vi "MQTT_Simple_Connect_and_Publish.vi"() -> ()   [LabVIEW 2018, in "MQTT_Functions.lvlib"]
uses:
  MQTT_Functions.lvlib
  Controls/QoS.ctl
  Controls/Retain_Flag.ctl
  Controls/DUP_Flag.ctl
  Controls/Connection_Return_Codes.ctl
  Controls/User_Info.ctl
  Controls/Connect_Flags.ctl
panel:
  in  "User Info":T1
  out "Message published":string
  in  "Stop Publishing":bool
  out "Message ID (acknowledged)":u16=10
  out "Acknowledged":bool
  in  "Message ID":u16=20
  in  "MQTT Broker":cluster{"address (IP)":string, "port":u16}={"address (IP)"="127.0.0.1", "port"=1883}
  in  "Message to be published":string="Quaxo says it's "
  out "Connection Status":T2=enum."Connection refused: not authorized"
  out "error out":errorcluster
  in  "Client ID":string="NodeE-12345"
  in  "error in (no error)":errorcluster
  in  "Topic":string[](array[string])
  in  "Publish Meta":cluster{"QoS":T3, "Retain":T4, "DUP":T5}
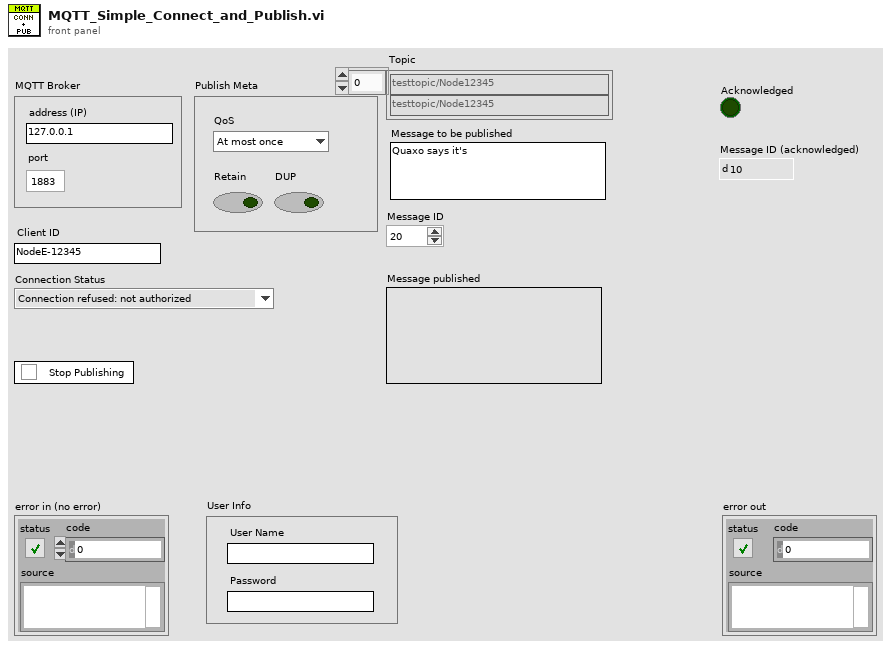
[diagram p1: front panel]
types:
  T1 = typedef "MQTT_Functions.lvlib/User_Info.ctl" = cluster{"User Name":string, "Password":string}
  T2 = typedef "MQTT_Functions.lvlib/Connection_Return_Codes.ctl" = enum16{"Connection accepted", "Connection refused: unacceptable protocol version", "Connection refused: identifier rejected", "Connection refused: Server unavailable", "Connection refused: bad user name or password", "Connection refused: not authorized"}
  T3 = typedef "MQTT_Functions.lvlib/QoS.ctl" = enum8{"At most once", "At least once", "Exactly once", "Reserved"}
  T4 = typedef "MQTT_Functions.lvlib/Retain_Flag.ctl" = bool
  T5 = typedef "MQTT_Functions.lvlib/DUP_Flag.ctl" = bool
  T6 = typedef "MQTT_Functions.lvlib/Connect_Flags.ctl" = cluster{"user name":bool, "password":bool, "will retain":bool, "will flag":bool, "clean session":bool, "reserved":bool, "will QoS":T3}
  T7 = cluster{"QoS":T3, "DUP":T5, "Retain":T4, "Keep Alive (sec)":u16}
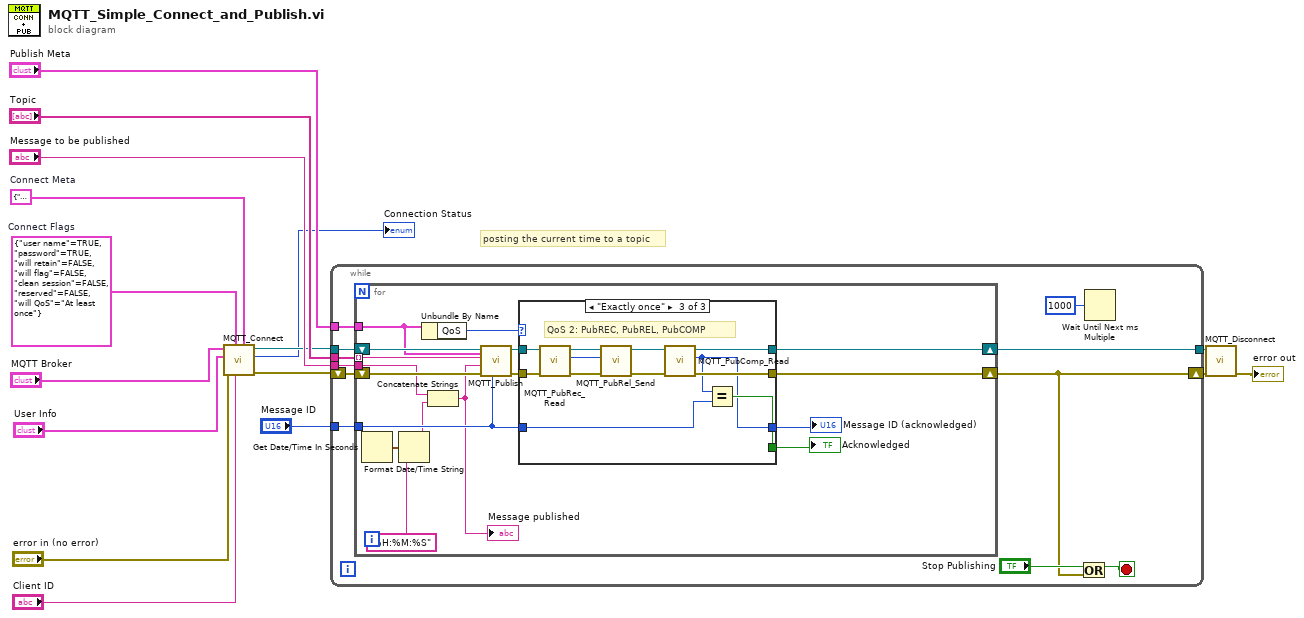
[diagram p0: block diagram]
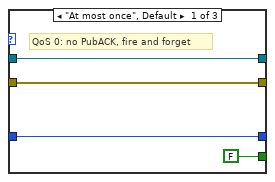
[diagram p2: hidden frame]
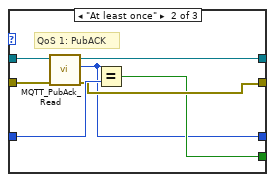
[diagram p3: hidden frame]
diagram:
  w14 = T6 {"user name"=TRUE, "password"=TRUE, "will retain"=FALSE, "will flag"=FALSE, "clean session"=FALSE, "reserved"=FALSE, "will QoS"=enum."At least once"}  # Connect Flags
  w11 = T7 {"QoS"=enum."At most once", "DUP"=FALSE, "Retain"=FALSE, "Keep Alive (sec)"=60}  # Connect Meta
  # "posting the current time to a topic"
  n1 = call "MQTT_Connect.vi"("Connect Meta"=w11, "Client ID"="Client ID", "Connect Flags"=w14, "error in (no error)"="error in (no error)", "User Info"="User Info", "MQTT Broker"="MQTT Broker") -> ("error out"=w2:errorcluster, "Connection Status"=→"Connection Status":T2, "connection ID out"=w4:refnum<k5>)  [unwired: 3 in]
  n2 = while {
    tunnel: "Topic" -> [w27]
    tunnel: "Message to be published" -> [w20]
    tunnel: w4 -> [w26]
    tunnel: "Publish Meta" -> [w24]
    tunnel: [w23] -> w7
    tunnel: "Message ID" -> [w22]
    shift-right: [w18] -> w8
    shift-left: w2 -> [w25]
    stop <- w19 stop-if-true
    n3 = for {
      tunnel: w27 -> [w44] mode=indexing
      tunnel: w24 -> [w41]
      tunnel: w22 -> [w36]
      tunnel: w20 -> [w35]
      shift-right: [w37] -> w23
      shift-left: w26 -> [w43]
      shift-right: [w30] -> w18
      shift-left: w25 -> [w42]
      n4 = Get Date/Time In Seconds() -> (seconds since 1Jan1904=w34:timestamp)
      n5 = Format Date/Time String(time format string (%c)="%H:%M:%S", seconds (now)=w34) -> (date/time string=w32:string)  [unwired: 1 in]
      n6 = Unbundle By Name(w41) -> ("QoS"=w40:T3)
      n7 = Concatenate Strings(w35, w32) -> (w31:string)
      "Message published" <- w31
      n8 = call "MQTT_Publish.vi"("Message ID"=w36, "Publish Meta"=w41, "error in (no error)"=w42, "Message to be published"=w31, "Topic"=w44, "connection ID"=w43) -> ("error out"=w39:errorcluster, "connection ID out"=w38:refnum<k5>)  [unwired: 4 in]
      n9 = case shown="\"Exactly once\"" w40 {
        tunnel: w39 -> [w47 w54 w66]
        tunnel: w38 -> [w48 w55 w67]
        tunnel: [w47 w52 w57] -> w30
        tunnel: [w48 w51 w58] -> w37
        tunnel: w36 -> [w45 w53 w65]
        tunnel: [FALSE w50 w59] -> w29
        tunnel: [w45 w49 w56] -> w28
        frame "At most once", Default {
          # "QoS 0: no PubACK, fire and forget"
        }
        frame "At least once" {
          # "QoS 1: PubACK"
          n10 = call "MQTT_PubAck_Read.vi"("error in (no error)"=w54, "connection ID"=w55) -> ("error out"=w52:errorcluster, "Message ID"=w49:u16, "connection ID out"=w51:refnum<k5>)  [unwired: 7 in]
          n11 = Equal?(x=w49, y=w53) -> (x = y?=w50:bool)
        }
        frame "Exactly once" {
          # "QoS 2: PubREC, PubREL, PubCOMP"
          n12 = call "MQTT_PubRec_Read.vi"("error in (no error)"=w66, "connection ID"=w67) -> ("error out"=w64:errorcluster, "Message ID"=w62:u16, "connection ID out"=w63:refnum<k5>)  [unwired: 7 in]
          n13 = call "MQTT_PubRel_Send.vi"("error in (no error)"=w64, "Message ID"=w62, "connection ID"=w63) -> ("error out"=w60:errorcluster, "connection ID out"=w61:refnum<k5>)  [unwired: 6 in, 1 out]
          n14 = call "MQTT_PubComp_Read.vi"("error in (no error)"=w60, "connection ID"=w61) -> ("error out"=w57:errorcluster, "Message ID"=w56:u16, "connection ID out"=w58:refnum<k5>)  [unwired: 7 in]
          n15 = Equal?(x=w56, y=w65) -> (x = y?=w59:bool)
        }
      }
      "Acknowledged" <- w29
      "Message ID (acknowledged)" <- w28
    }
    n16 = Or(x="Stop Publishing", y=w18) -> (x .or. y?=w19:bool)
    n17 = Wait Until Next ms Multiple(millisecond multiple=u32 1000) -> ()  [unwired: 1 out]
  }
  n18 = call "MQTT_Disconnect.vi"("error in (no error)"=w8, "connection ID"=w7) -> ("error out"=→"error out":errorcluster)  [unwired: 9 in]
